vi "Measure.vi"(6 "error in (no error)":errorcluster, 9 "Abstract Sensor in":refnum<class "Abstract Sensor.lvclass">) -> (0 "error out":errorcluster, 2 "Array of Measurement":dbl[](array[numeric]), 3 "Abstract Sensor out":refnum<class "Abstract Sensor.lvclass">)   [LabVIEW 2014, in "Abstract Sensor.lvlib" / "Abstract Sensor.lvclass"]
uses:
  Abstract Sensor.lvclass
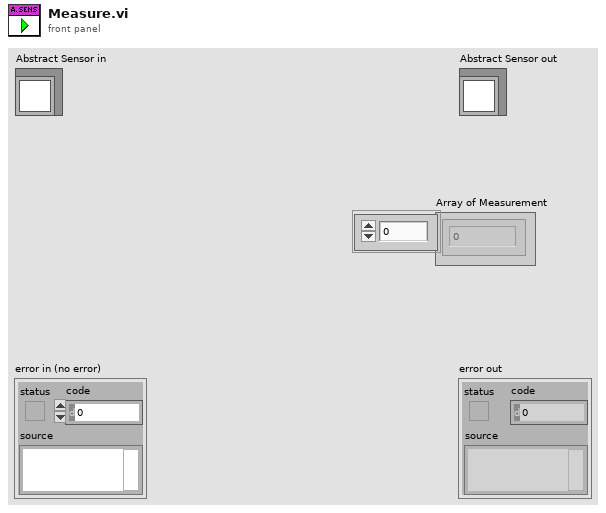
[diagram p1: front panel]
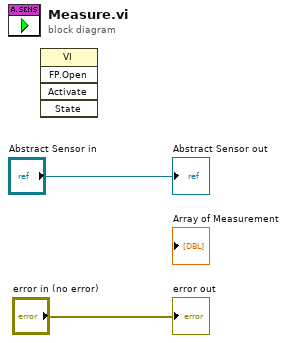
[diagram p0: block diagram]
diagram:
  n1 = invoke class="VI" method="FP.Open"() -> ()  [unwired: 5 in, 5 out]
  "error out" <- "error in (no error)"
  "Abstract Sensor out" <- "Abstract Sensor in"
